vi "binary_as_string.vi"() -> ()   [LabVIEW 2021]
panel:
  out "path":path
  out "text":string
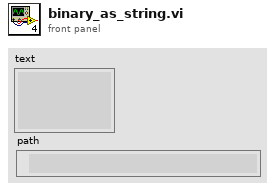
[diagram p1: front panel]
types:
  T1 = enum16{"open", "replace", "create", "open or create", "replace or create", "replace or create with confirmation"}
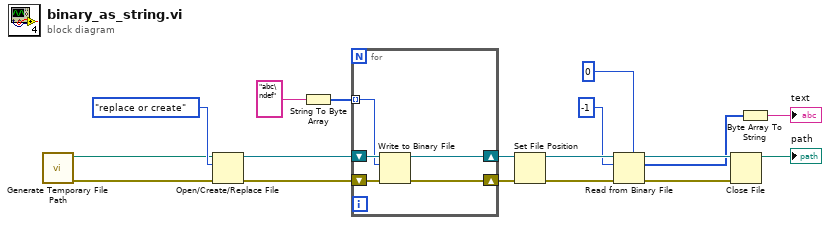
[diagram p0: block diagram]
diagram:
  n1 = call <vilib>:"Generate Temporary File Path.vi"() -> ("error out"=w17:errorcluster, "Unique Temporary File Path"=w16:path)  [unwired: 10 in]
  n2 = Open/Create/Replace File(file path (use dialog)=w16, error in=w17, operation (0:open)=T1."replace or create") -> (refnum out=w15:refnum<file>, error out=w13:errorcluster)  [unwired: 3 in, 1 out]
  n3 = String To Byte Array(string="abc\ndef") -> (unsigned byte array=w5:u8[])
  n4 = for {
    shift-right: [w22] -> w14
    shift-left: w15 -> [w23]
    shift-right: [w20] -> w12
    shift-left: w13 -> [w21]
    tunnel: w5 -> [w19] mode=indexing
    n5 = Write to Binary File(file (use dialog)=w23, data=w19, error in=w21) -> (refnum out=w22:refnum<file>, error out=w20:errorcluster)  [unwired: 3 in, 1 out]
  }
  n6 = Set File Position(refnum=w14, error in=w12) -> (refnum out=w11:refnum<file>, error out=w10:errorcluster)  [unwired: 2 in]
  n7 = Read from Binary File(5:u8 0, 8:w10, 10:-1 ("count (1)"), 11:w11) -> (0:w9:errorcluster, 2:w3:u8[], 3:w8:refnum<file>)  [unwired: 2 in, 1 out]
  n8 = Close File(refnum=w8, error in=w9) -> (path=→"path":path)  [unwired: 1 out]
  n9 = Byte Array To String(unsigned byte array=w3) -> (string=→"text":string)
